vi "Generate Data Clusters.vi"(8 "error in (no error)":errorcluster, 11 "Item Ref in":T1 format="%.0x") -> (0 "error out":errorcluster, 1 "Outputs":T8, 2 "Inputs":T9, 3 "Parent Ref out":T1 format="%.0x", 4 "Input References":T7 {"Input Registers" format="%.0x"; "Discrete Inputs" format="%.0x"})   [LabVIEW 2015]
uses:
  <vilib>/NI Veristand/Custom Device API/Custom Device Item Ref.ctl
  Shared/Controls/Data Model/Input Channel Data.ctl
  Shared/Controls/Data Model/Channel.ctl
  Modbus Type.ctl
  Shared/Controls/Data Model/Mapping.ctl
  Shared/Controls/Data Model/DataType.ctl
  Shared/Controls/Data Model/Output Channel Data.ctl
  Shared/Controls/Data Model/Input References.ctl
  Shared/Controls/Data Model/Output References.ctl
  Modbus Master System Explorer.lvlib
  Shared/Modbus Master Shared.lvlib
  <vilib>/NI VeriStand/Custom Device API/Custom Device API.lvlib
panel:
  in  "Start Index":i32
  out "Channel Registers":T1[](array[typedef]) format="%.0x"
  out "End Index":i32
  out "Channels":T2[](array[typedef])
  in  "Type":T3
  out "Output References":T6 {"Holding Registers" format="%.0x"; "Coils" format="%.0x"}
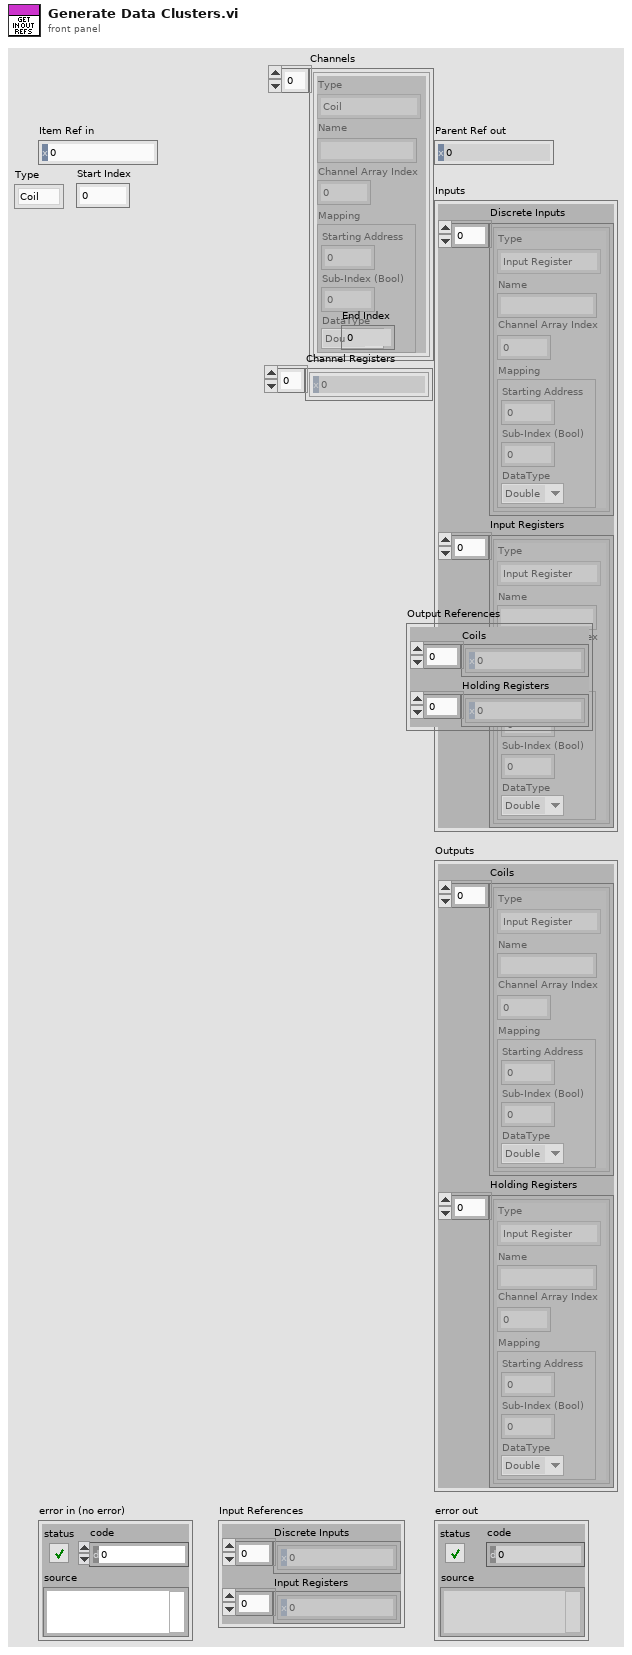
[diagram p1: front panel]
types:
  T1 = typedef "Custom Device API.lvlib/Custom Device Item Ref.ctl" = u64
  T2 = typedef "Modbus Master Shared.lvlib/Channel.ctl" = cluster{"Type":T3, "Name":string, "Channel Array Index":i32, "Mapping":T4}
  T3 = typedef "Modbus Master Shared.lvlib/Modbus Type.ctl" = enum16{"Coil", "Discrete Input", "Holding Register", "Input Register"}
  T4 = typedef "Modbus Master Shared.lvlib/Mapping.ctl" = cluster{"Starting Address":u16, "Sub-Index (Bool)":u16, "DataType":T5}
  T5 = typedef "Modbus Master Shared.lvlib/DataType.ctl" = enum16{"Double", "Single", "I64", "I32", "I16", "I8", "U64", "U32", "U16", "U8", "Boolean"}
  T6 = typedef "Modbus Master Shared.lvlib/Output References.ctl" = cluster{"Coils":T1[], "Holding Registers":T1[]}
  T7 = typedef "Modbus Master Shared.lvlib/Input References.ctl" = cluster{"Discrete Inputs":T1[], "Input Registers":T1[]}
  T8 = typedef "Modbus Master Shared.lvlib/Output Channel Data.ctl" = cluster{"Coils":T2[], "Holding Registers":T2[]}
  T9 = typedef "Modbus Master Shared.lvlib/Input Channel Data.ctl" = cluster{"Discrete Inputs":T2[], "Input Registers":T2[]}
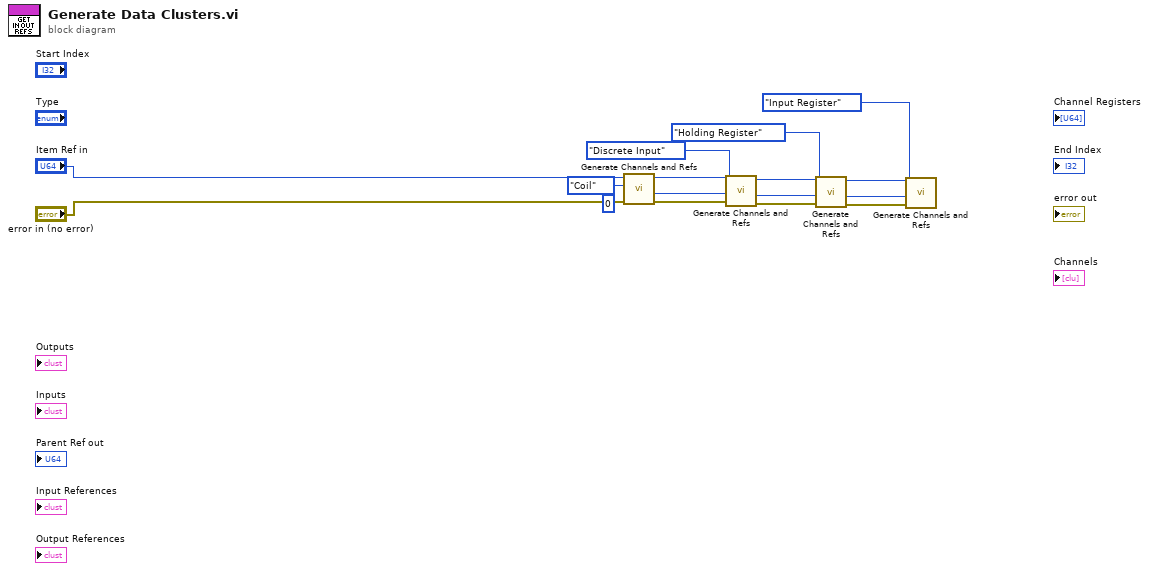
[diagram p0: block diagram]
diagram:
  n1 = call "Generate Channels and Refs.vi"("error in (no error)"="error in (no error)", "Start Index in"=0, "Type"=Modbus_Type."Coil", "Item Ref in"="Item Ref in") -> ("error out"=w5:errorcluster, "Next Index"=w12:i32, "Item Ref out"=w7:T1)  [unwired: 3 in, 2 out]
  n2 = call "Generate Channels and Refs.vi"("error in (no error)"=w5, "Start Index in"=w12, "Type"=Modbus_Type."Discrete Input", "Item Ref in"=w7) -> ("error out"=w9:errorcluster, "Next Index"=w6:i32, "Item Ref out"=w10:T1)  [unwired: 3 in, 2 out]
  n3 = call "Generate Channels and Refs.vi"("error in (no error)"=w9, "Start Index in"=w6, "Type"=Modbus_Type."Holding Register", "Item Ref in"=w10) -> ("error out"=w4:errorcluster, "Next Index"=w3:i32, "Item Ref out"=w2:T1)  [unwired: 3 in, 2 out]
  n4 = call "Generate Channels and Refs.vi"("error in (no error)"=w4, "Start Index in"=w3, "Type"=Modbus_Type."Input Register", "Item Ref in"=w2) -> ()  [unwired: 3 in, 5 out]
